vi "Panel Resized.vi"(6 "Sizing Refnums":T2, 8 "error in (no error)":errorcluster, 9 "Origin":cluster{"H":i16, "V":i16}, 10 "NewBnds":T1, 11 "Size Constraints":cluster{"min tab width":i32, "w/h":dbl}) -> (0 "error out":errorcluster)   [LabVIEW 2017]
uses:
  <vilib>/Utility/miscctls.llb/LVRectTypeDef.ctl
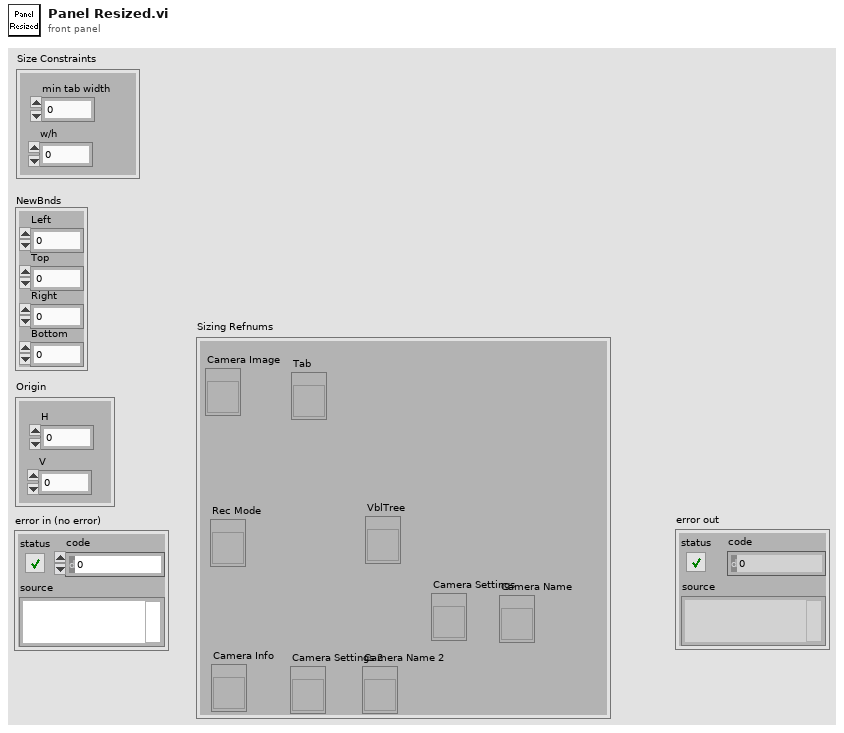
[diagram p1: front panel]
types:
  T1 = typedef "LVRectTypeDef.ctl" = cluster{"Left":i16, "Top":i16, "Right":i16, "Bottom":i16}
  T2 = cluster{"Camera Image":refnum<vi>, "Tab":refnum<vi>, "Rec Mode":refnum<vi>, "VblTree":refnum<vi>, "Camera Settings":refnum<vi>, "Camera Name":refnum<vi>, "Camera Info":refnum<vi>, "Camera Settings 2":refnum<vi>, "Camera Name 2":refnum<vi>}
  T3 = typedef "LVPositionTypeDef.ctl" = cluster{"Left":i32, "Top":i32}
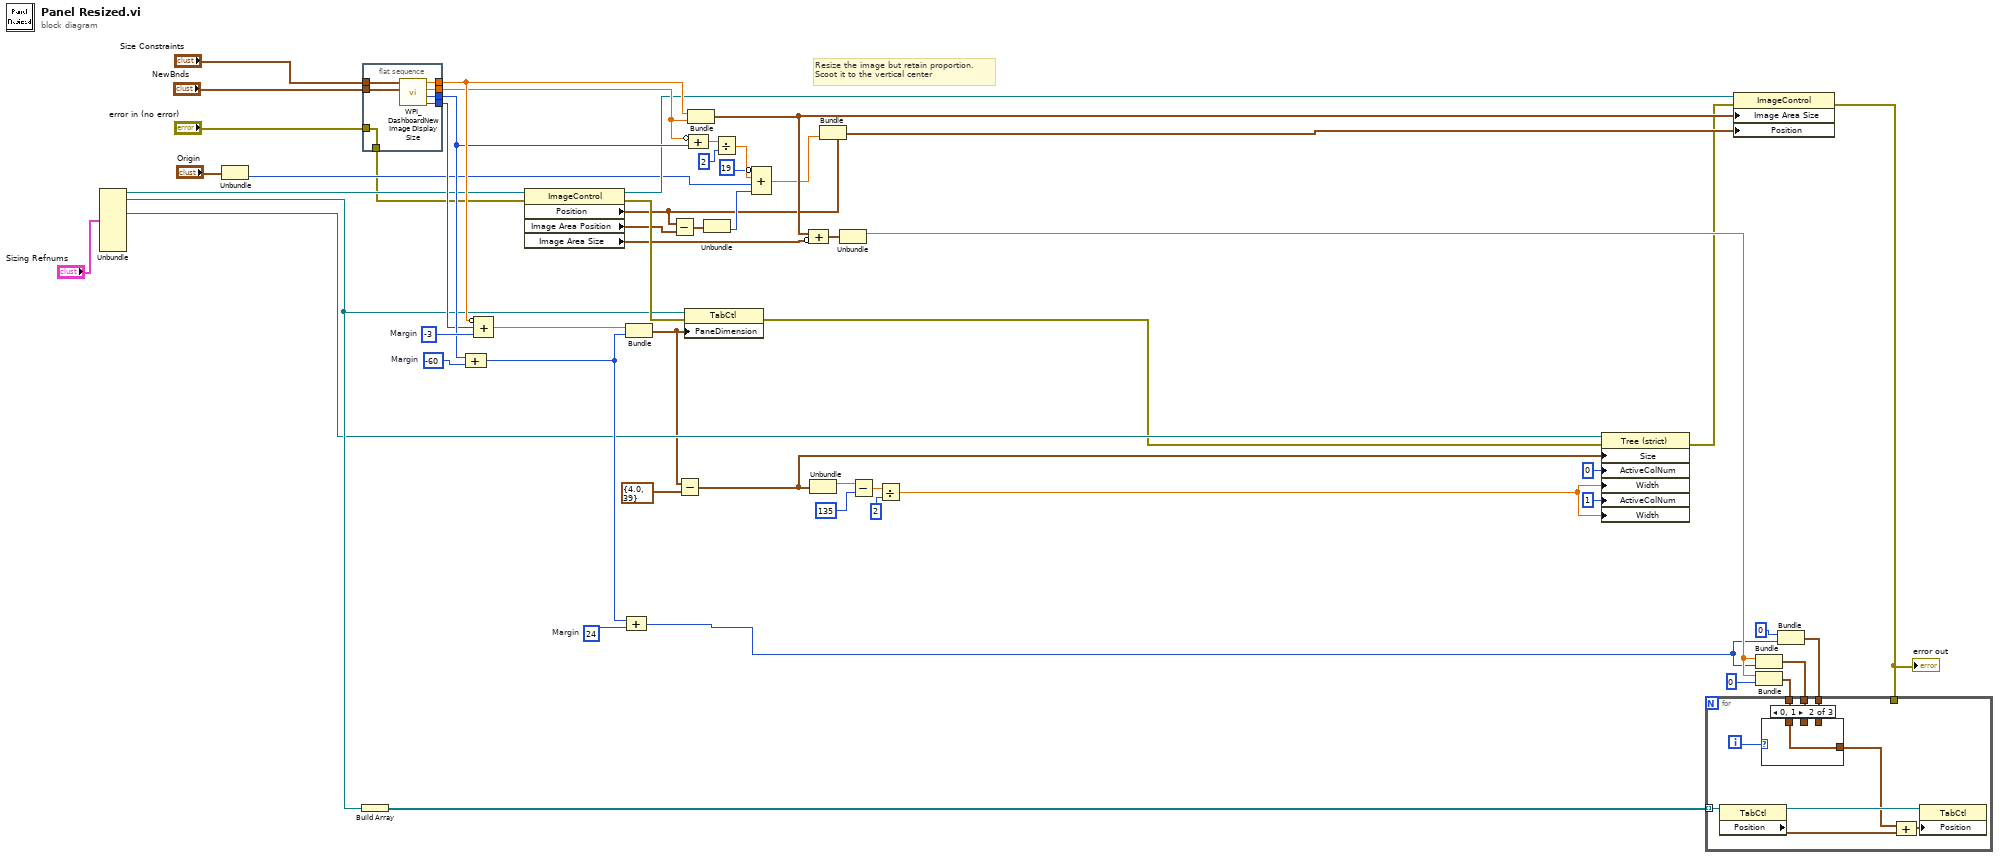
[diagram p0: block diagram]
diagram:
  w47 = 24  # Margin
  w44 = -60  # Margin
  w51 = -3  # Margin
  # "Resize the image but retain proportion.\nScoot it to the vertical center"
  n1 = Unbundle("Sizing Refnums") -> ("Camera Image"=w19:refnum<vi>, "Tab"=w20:refnum<vi>, "VblTree"=w11:refnum<vi>)  [unwired: 6 out]
  n2 = Unbundle("Origin") -> ("V"=w25:i16)  [unwired: 1 out]
  n3 = Build Array(w20) -> (w55:refnum<vi>[])
  n4 = flat-sequence {
    tunnel: "NewBnds" -> [w62]
    tunnel: "Size Constraints" -> [w61]
    tunnel: [w60] -> w43
    tunnel: [w59] -> w48
    tunnel: [w58] -> w49
    tunnel: [w57] -> w50
    tunnel: [w56] -> w15
    tunnel: "error in (no error)" -> [w56]
    frame #0 {
      n5 = call <vilib>:"WPI_DashboardNew Image Display Size.vi"("NewBnds"=w62, "Size Constraints"=w61) -> ("Window Width"=w60:i16, "Window Height"=w58:i16, "Height"=w59:dbl, "Width"=w57:dbl)  [unwired: 6 in]
    }
  }
  n6 = Compound Arithmetic op=unknown(w49, w44) -> (w46:i32)
  n7 = Compound Arithmetic op=ADD(invert w50, w43, w51) -> (w45:dbl)
  n8 = property class="ImageControl"(reference=w19, error in=w15) -> (reference out=w36:refnum<vi>, error out=w54:errorcluster, "Position"=w35:T3, "Image Area Position"=w30:cluster{"Left":i32, "Top":i32}, "Image Area Size"=w41:cluster{"Width":u32, "Height":u32})
  n9 = Bundle(w45, w46) -> (w7:cluster{dbl, i32})  [unwired: 1 in]
  n10 = Compound Arithmetic op=ADD(w46, w47) -> (w14:i32)
  n11 = Subtract(x=w35, y=w30) -> (x-y=w37:T3)
  n12 = Subtract(x=w7, y=cluster{dbl, i32} {4.0, 39}) -> (x-y=w2:cluster{dbl, i32})
  n13 = property class="TabCtl"(reference=w20, error in=w54, "PaneDimension"=w7) -> (error out=w10:errorcluster)  [unwired: 1 out]
  n14 = Bundle("Width"=w50, "Height"=w48) -> (w39:cluster{"Width":dbl, "Height":dbl})  [unwired: 1 in]
  n15 = Compound Arithmetic op=ADD(invert w48, w49) -> (w31:dbl)
  n16 = Unbundle(w37) -> ("Top"=w38:i32)  [unwired: 1 out]
  n17 = Divide(x=w31, y=2) -> (x/y=w33:dbl)
  n18 = Compound Arithmetic op=ADD(invert 19, w33, w25, w38) -> (w34:dbl)
  n19 = Compound Arithmetic op=ADD(w39, invert w41) -> (w42:cluster{"Width":dbl, "Height":dbl})
  n20 = Unbundle(w2) -> (w6:dbl)  [unwired: 1 out]
  n21 = Bundle(cluster=w35, "Top"=w34) -> (w40:T3)  [unwired: 1 in]
  n22 = Unbundle(w42) -> ("Width"=w52:dbl)  [unwired: 1 out]
  n23 = Subtract(x=w6, y=135 ("Active Cell:Active Column Number")) -> (x-y=w4:dbl)
  n24 = Divide(x=w4, y=2 ("Active Cell:Active Column Number")) -> (x/y=w1:dbl)
  n25 = property class="Tree (strict)"(reference=w11, error in=w10, "Size"=w2, "ActiveColNum"=0 ("Active Cell:Active Column Number"), "Width"=w1, "ActiveColNum"=1 ("Active Cell:Active Column Number"), "Width"=w1) -> (error out=w9:errorcluster)  [unwired: 1 out]
  n26 = property class="ImageControl"(reference=w36, error in=w9, "Image Area Size"=w39, "Position"=w40) -> (error out=w24:errorcluster)  [unwired: 1 out]
  "error out" <- w24
  n27 = Bundle("Width"=w52, w14) -> (w29:cluster{"Width":dbl, i32})  [unwired: 1 in]
  n28 = Bundle("Width"=w52, 0) -> (w28:cluster{"Width":dbl, i32})  [unwired: 1 in]
  n29 = Bundle(0, w14) -> (w17:cluster{i32, i32})  [unwired: 1 in]
  n30 = for {
    tunnel: w55 -> [w71] mode=indexing
    tunnel: w29 -> [w65]
    tunnel: w28 -> [w66]
    tunnel: w24 -> [_]
    tunnel: w17 -> [w64]
    i -> [w67]
    n31 = property class="TabCtl"(reference=w71) -> (reference out=w70:refnum<vi>, "Position"=w69:T3)  [unwired: 1 in, 1 out]
    n32 = case shown="0, 1" w67 {
      tunnel: w66 -> [_ w73 _]
      tunnel: w65 -> [_ _ w74]
      tunnel: w64 -> [w72 _ _]
      tunnel: [w72 w73 w74] -> w63
      frame Default {
      }
      frame 0, 1 {
      }
      frame 2..4 {
      }
    }
    n33 = Compound Arithmetic op=ADD(w63, w69) -> (w68:cluster{dbl, i32})
    n34 = property class="TabCtl"(reference=w70, "Position"=w68) -> ()  [unwired: 1 in, 2 out]
  }
